vi "checkout_tlc.vi"(6 "destroy queue?":bool, 7 "locked by?":string, 8 "error in (no error)":errorcluster, 11 "GenericToplevelComponent in":refnum<class "GenericToplevelComponent.lvclass">) -> (0 "error out":errorcluster, 3 "GenericToplevelComponent out":refnum<class "GenericToplevelComponent.lvclass">)   [LabVIEW 2010, in "GenericToplevelComponent.lvclass"]
uses:
  GenericToplevelComponent.lvclass
  GenericToplevelComponent.lvclass/GenericToplevelComponent.ctl
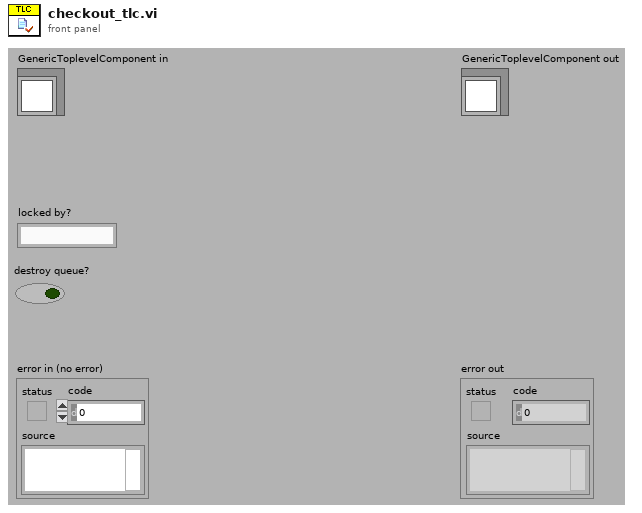
[diagram p1: front panel]
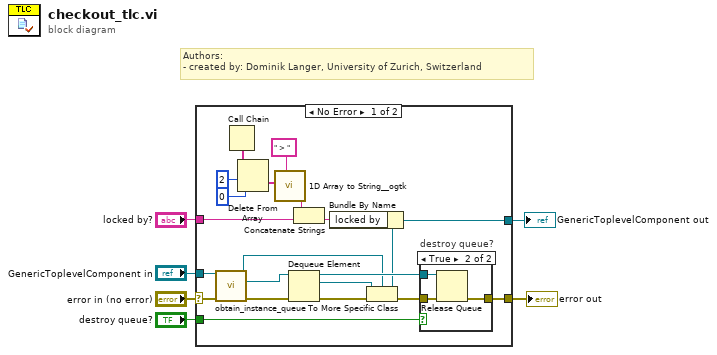
[diagram p0: block diagram]
diagram:
  # "Authors: \n- created by: Dominik Langer, University of Zurich, Switzerland"
  n1 = case shown="No Error" "error in (no error)" {
    selector: "error in (no error)" -> [w16 w33]
    tunnel: [w19 w33] -> w1
    tunnel: [w12 w32] -> w2
    tunnel: "GenericToplevelComponent in" -> [w13 w32]
    tunnel: "locked by?" -> [w27 _]
    tunnel: "destroy queue?" -> [w17 _]
    frame No Error {
      n2 = call-dynamic "obtain_instance_queue.vi"("error in (no error)"=w16, "GenericToplevelComponent in"=w13) -> ("error out"=w15:errorcluster, "instance queue"=w14:refnum<queue>, "GenericToplevelComponent out"=w11:refnum<class "GenericToplevelComponent.lvclass">)  [unwired: 7 in]
      n3 = Call Chain() -> (call chain=w21:string[])
      n4 = Delete From Array(array=w21, length=2, index=0) -> (array with subset deleted=w24:string[])  [unwired: 1 out]
      n5 = call <userlib>:"1D Array to String__ogtk.vi"("delimiter (Tab)"=" > ", "Array of Strings"=w24) -> ("delimited string"=w26:string)  [unwired: 9 out]
      n6 = Dequeue Element(queue=w14, error in (no error)=w15) -> (queue out=w18:refnum<queue>, element=w10:refnum<class "GenericComponent.lvclass">, error out=w8:errorcluster)  [unwired: 2 out]
      n7 = Concatenate Strings(w26, w27) -> (w20:string)
      n8 = To More Specific Class(target class=w11, reference=w10, error in=w8) -> (specific class reference=w9:refnum<class "GenericToplevelComponent.lvclass">, error out=w7:errorcluster)
      n9 = Bundle By Name(cluster=w9, "locked by"=w20) -> (w12:refnum<class "GenericToplevelComponent.lvclass">)
      n10 = case "destroy queue?" shown="True" w17 {
        tunnel: w7 -> [w28 w31]
        tunnel: [w28 w30] -> w19
        tunnel: w18 -> [_ w29]
        frame False {
        }
        frame True {
          n11 = Release Queue(queue=w29, error in (no error)=w31) -> (error out=w30:errorcluster)  [unwired: 1 in, 2 out]
        }
      }
    }
    frame Error {
    }
  }
  "error out" <- w1
  "GenericToplevelComponent out" <- w2
